vi "GetAttributeViReal64_SA-Marker_Source.vi"(8 "error in (no error)":errorcluster {"code" format="%.0x"}, 9 "AttributeID":u32(ring)=1150712 items=["SA_MARKER_AMPLITUDE"=1150712, "SA_MARKER_FREQUENCYCOUNTER_GATE_TIME"=1150683, "SA_MARKER_FUNCTION_BAND_LEFT"=1150693, "SA_MARKER_FUNCTION_BAND_RIGHT"=1150694, "SA_MARKER_FUNCTION_BAND_SPAN"=1150695, "SA_MARKER_NDBPOINTS_RESULTS"=1150688, "SA_MARKER_NDBPOINTS_VALUE"=1150687, "SA_MARKER_PEAK_EXCURSION"=1150714, "SA_MARKER_POSITION"=1150715, "SA_MARKER_REFERENCE_AMPLITUDE"=1150716, "SA_MARKER_REFERENCE_POSITION"=1150717, "SA_MARKER_THRESHOLD"=1150719, "SA_MARKER_X_AXIS_TRACE_POINTS"=1150710, "SA_MARKER_Y"=1150702, "SA_SOURCE_FREQUENCY_OFFSET"=1150797, "SA_SOURCE_LEVEL_AMPLITUDE"=1150785, "SA_SOURCE_LEVEL_AMPLITUDE_OFFSET"=1150790, "SA_SOURCE_LEVEL_AMPLITUDE_STEP"=1150791, "SA_SOURCE_LEVEL_POWER_SWEEP"=1150788, "SA_SOURCE_LEVEL_TRACK_DELAY"=1150793], 11 "instrument handle":refnum<k15>) -> (0 "error out":errorcluster {"code" format="%.0x"}, 2 "AttributeValue":dbl, 3 "instrument handle out":refnum<k15>)   [LabVIEW 2009, in "Keysight XSAn.lvlib"]
doc: "Gets a Real64 attribute from the instrument driver.\nThe following Attributes are supported:\n\nSA_MARKER_AMPLITUDE\nSA_MARKER_FREQUENCYCOUNTER_GATE_TIME\nSA_MARKER_FUNCTION_BAND_LEFT\nSA_MARKER_FUNCTION_BAND_RIGHT\nSA_MARKER_FUNCTION_BAND_SPAN\nSA_MARKER_NDBPOINTS_RESULTS\nSA_MARKER_NDBPOINTS_VALUE\nSA_MARKER_PEAK_EXCURSION\nSA_MARKER_POSITION\nSA_MARKER_REFERENCE_AMPLITUDE\nSA_MARKER_REFERENCE_POSITION\nSA_MARKER_THRESHOLD\nSA_MARKER_X_AXIS_TRACE_POINTS\nSA_MARKER_Y\nSA_SOURCE_FREQUENCY_OFFSET\nSA_SOURCE_LEVEL_AMPLITUDE\nSA_SOURCE_LEVEL_AMPLITUDE_OFFSET\nSA_SOURCE_LEVEL_AMPLITUDE_STEP\nSA_SOURCE_LEVEL_POWER_SWEEP\nSA_SOURCE_LEVEL_TRACK_DELAY"
uses:
  <instrlib>/Keysight XSAn/Keysight XSAn.lvlib
  AgXSAn.dll
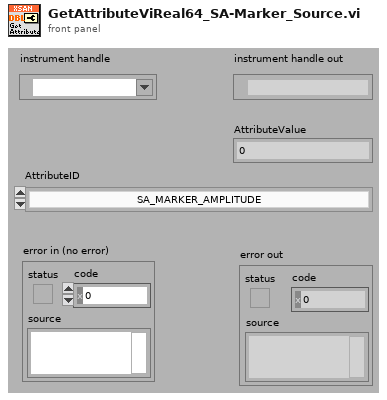
[diagram p1: front panel]
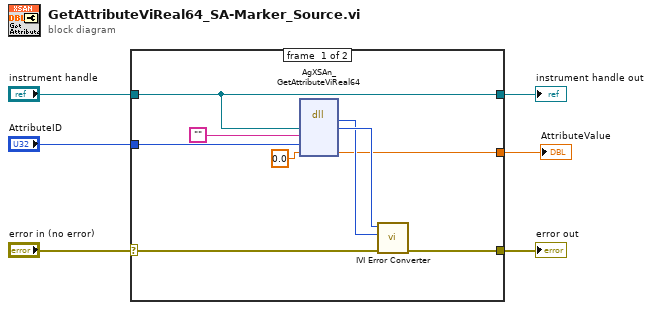
[diagram p0: block diagram]
diagram:
  n1 = case shown="No Error" "error in (no error)" {
    selector: "error in (no error)" -> [w13 w17]
    tunnel: [w12 w17] -> w6
    tunnel: "instrument handle" -> [w8 w16]
    tunnel: "AttributeID" -> [w11 _]
    tunnel: [w9 _] -> w2
    tunnel: [w8 w16] -> w1
    frame #0 {
      n2 = dll-call lib="AgXSAn**.dll" fn="AgXSAn_GetAttributeViReal64"("Vi"=w8, "RepCapIdentifier"="", "AttributeID"=w11, "AttributeValue"=0.0) -> ("return type"=w14:i32, "Vi"=w15:u32, "AttributeValue"=w9:dbl)  [unwired: 5 in, 2 out]
      n3 = call <instrlib>:"IVI Error Converter.vi"("error in (no error)"=w13, "IVI error code (0)"=w14, "instrument handle"=w15) -> ("error out"=w12:errorcluster)  [unwired: 7 in, 1 out]
    }
    frame #1 {
    }
  }
  "error out" <- w6
  "instrument handle out" <- w1
  "AttributeValue" <- w2
